vi "bez_daq.vi"() -> ()   [LabVIEW 2019, in "Main.lvlib"]
doc: "Main VI program. \n1. After starting the program, click PowerUP to turn on the calibrator.\n2. The program in Standby can pick the signal values with the use of the keyboard or SetUP mode. \nThe SetUP VI can configure can change the signal type, offset and phase. \n3. Click Operate to go to Operate mode. First 2 Warning message will be shown, then the program will start with Operate mode.\n4. Click Standby to go to standby again, then the program will stop with the DaQ and Operating mode.\n5. Click PowerUP to sotp the program"
uses:
  Main.lvlib
  Tipski Definicii/Kalibrator_Sostojbi.ctl
  Signal/Signal.lvlib
  Tipski Definicii/Keyboard_Sostojbi.ctl
  subVIS/Main_Programs_SubVIs.lvlib
  Tipski Definicii/QMH_Daq_States.ctl
  Polymorphic/Queues.lvlib
  Polymorphic/Enq_DaQ_QMH.vi
  Polymorphic/Enq_Calibrator_QMH.vi
  Polymorphic/Prev_Calibrator_QMH.vi
  Tipski Definicii/check.ctl
  Tipski Definicii/error_handl.ctl
  Tipski Definicii/Signal Values.ctl
  Tipski Definicii/rel_error.ctl
  Tipski Definicii/danger.ctl
  Tipski Definicii/Unit.ctl
  Polymorphic/DeQ_Calibrator_QMH.vi
  Polymorphic/Init_Main.vi
  Polymorphic/Release_Main.vi
  Polymorphic/DaQ_Signal.vi
panel:
  out "AuxA":bool
  out "NormalV":bool
  in  "Knob":dbl(knob) scale=-3.0..3.0 scale format="%#.3g"
  out "Lev_Indikator":string
  out "Desen_Indikator":string
  out "Scope Out":bool
  out "Scope In":bool
  out "AuxAOut":bool
  out "NormalVOut":bool
  in  "V":bool
  in  "Trig":bool
  in  "Tocka":bool
  in  "0":bool
  in  "STBY":bool
  in  "Shift":bool
  in  "SetUP":bool
  in  "Scope":bool
  in  "Save":bool
  in  "Reset":bool
  in  "Power Up":bool
  in  "Plus":bool
  in  "Opr":bool
  in  "Ohm":bool
  in  "NewRef":bool
  in  "Multi":bool
  in  "Meas":bool
  in  "M":bool
  in  "k":bool
  in  "Hz":bool
  in  "F":bool
  in  "Enter":bool
  in  "Earth":bool
  in  "Div":bool
  in  "Conn?":bool
  in  "CE":bool
  in  "C":bool
  in  "Boost":bool
  in  "A":bool
  in  "9":bool
  in  "m":bool
  in  "8":bool
  in  "7":bool
  in  "6":bool
  in  "5":bool
  in  "4":bool
  in  "3":bool
  in  "2":bool
  in  "1":bool
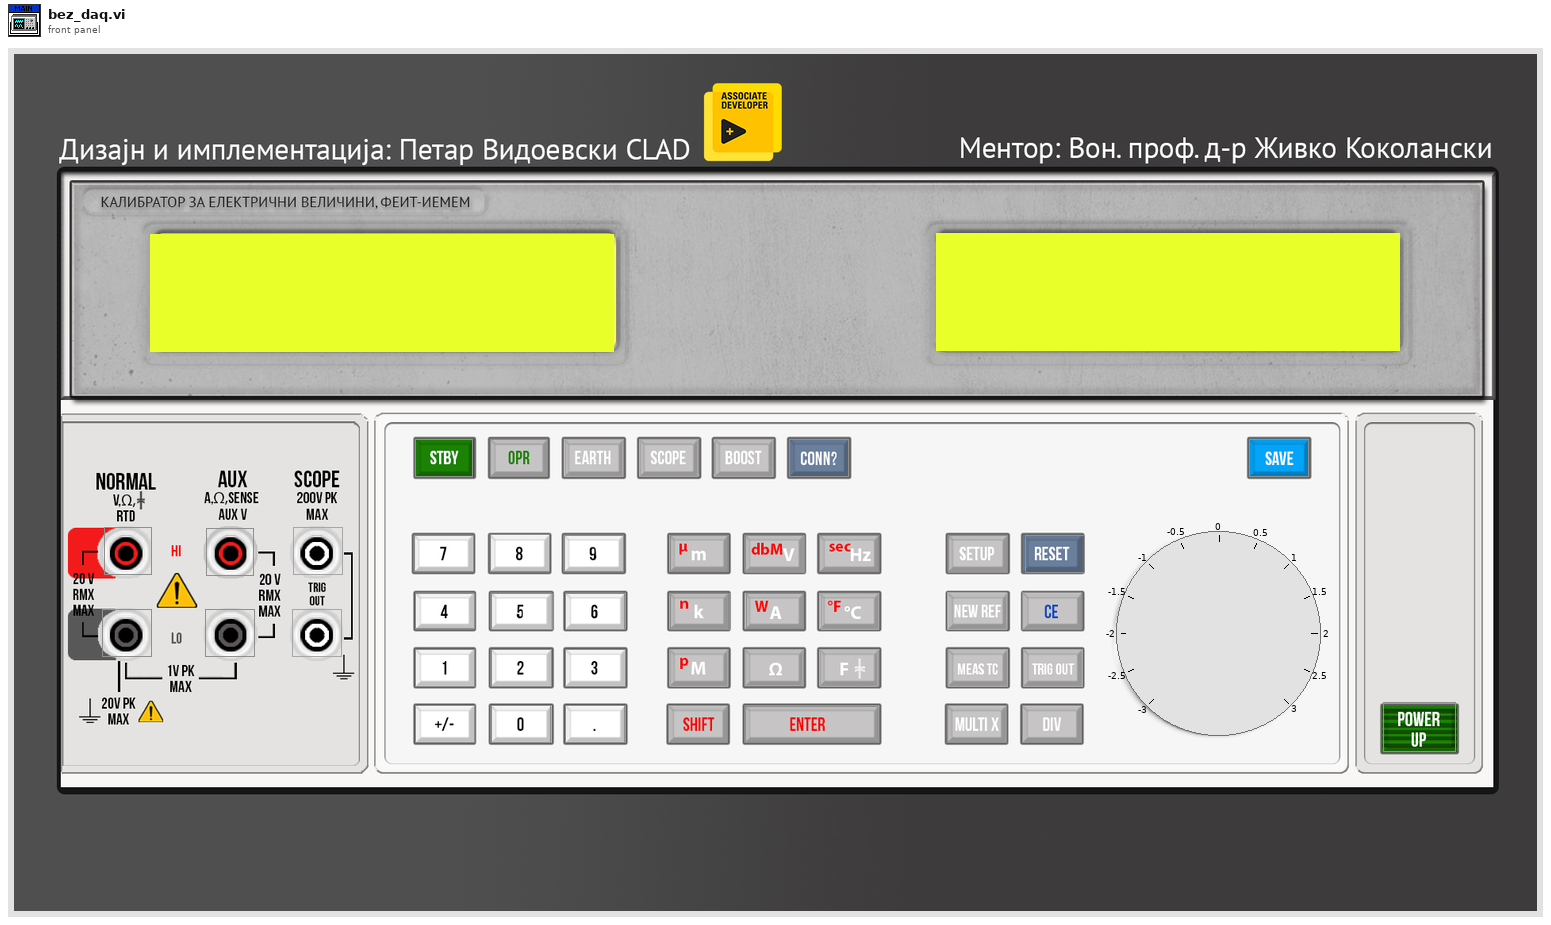
[diagram p1: front panel]
types:
  T1 = cluster{"Calibrator Queue ":refnum<queue>, "ER Refnum":refnum<event-registration>, "User Event in":refnum<user-event>, "QMH Queue ":refnum<queue>, "DaQ Notifier":refnum<notifier>}
  T2 = typedef "Main_program_queues.ctl" = cluster{"Calibrator QMH":refnum<queue>, "DaQ QMH":refnum<queue>, "DaQ":refnum<queue>, "ER":refnum<event-registration>, "User Event":refnum<user-event>}
  T3 = typedef "error_handl.ctl" = enum16{"Init", "Insert Error 1", "Insert Error 2", "Insert Error 3", "Insert Error 4", "Handle Erros"}
  T4 = enum16{"Init", "Init DaQ", "Start", "Output", "Stop", "Delete", "V/A ?"}
  T5 = typedef "Unit.ctl" = enum16{"Init", "Add", "Read"}
  T6 = typedef "rel_error.ctl" = enum16{"Init", "Add String", "Error", "Get Error and Strings", "Reset"}
  T7 = typedef "danger.ctl" = enum16{"Init", "Check"}
  T8 = typedef "check.ctl" = enum16{"Init", "Add dot", "Add +", "Add Shift", "Check", "Reset", "Reset Shift"}
  T9 = typedef "Signal Values.ctl" = enum16{"Init", "Add V/A string", "Add Hz string", "Get Strings and Values", "Reset", "Add Offset", "Add Waveform", "Add Phase"}
  T10 = typedef "Kalibrator_Sostojbi.ctl" = enum16{"Init", "Idle", "Standby", "Operate ", "End"}
  T11 = typedef "Keyboard_Sostojbi.ctl" = enum16{"Init", "Add Number", "Add Decimal", "Add Unit ", "Clear", "Read", "Enter", "CE", "Add Unit Scale", "Check Unit", "Mul", "Div"}
  T12 = cluster{"Amp String":string, "Amp Value":dbl, "Hz Value Out":dbl, "Waveform Out":enum16{"Sine Wave", "Triangle Wave", "Square Wave", "Sawtooth Wave"}, "Offset Out":dbl, "Phase Out":dbl, "Signal String":string, "Signal":waveform(dbl)}
  T13 = cluster{"Voltage":bool, "Current":bool, "Scope":bool}
  T14 = typedef "QMH_Daq_States.ctl" = enum16{"Idle", "Start DaQ", "DaQ", "Generate Message", "Stop DaQ", "End"}
  T15 = enum32{"Invalid", "Standard", "Closed", "Hidden", "Minimized", "Maximized"}
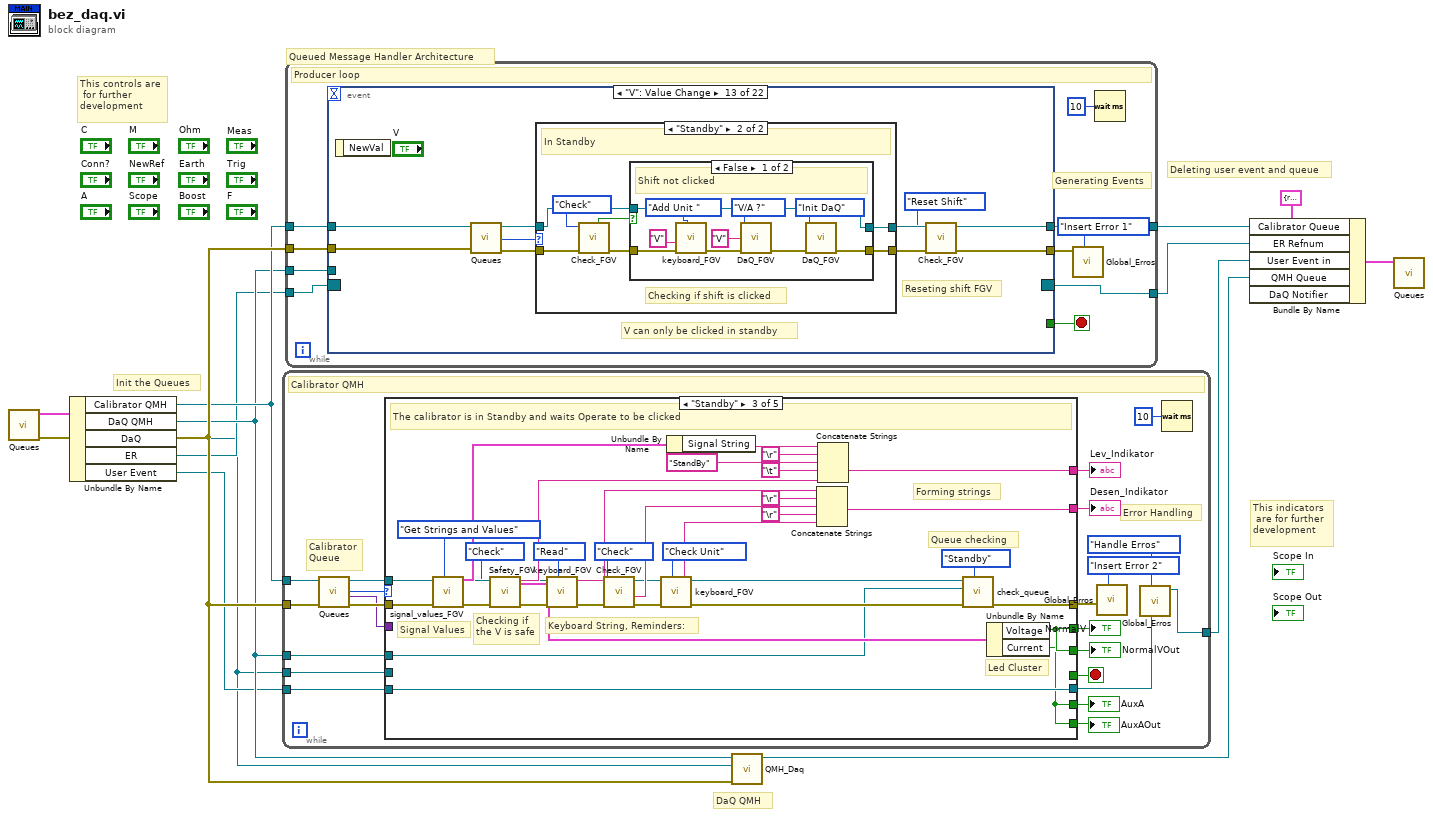
[diagram p0: block diagram]
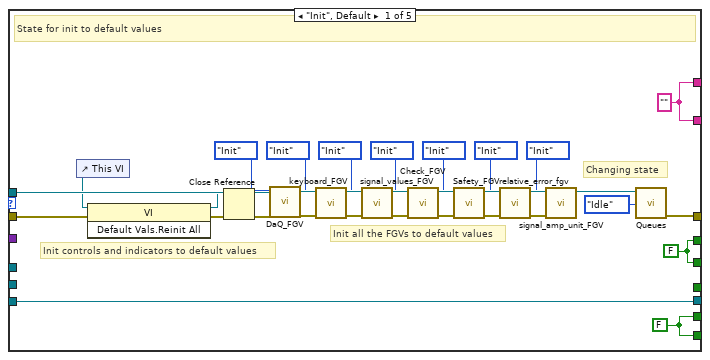
[diagram p2: hidden frame]
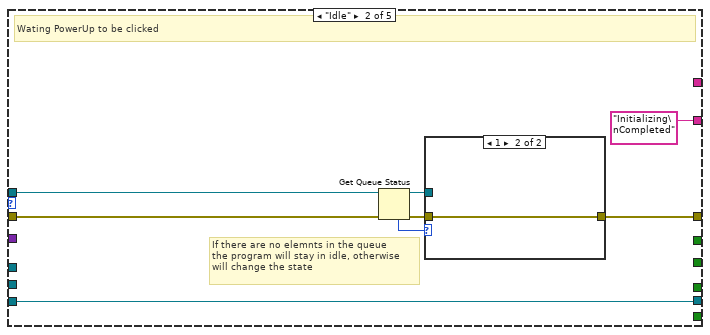
[diagram p3: hidden frame]
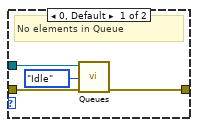
[diagram p4: hidden frame]
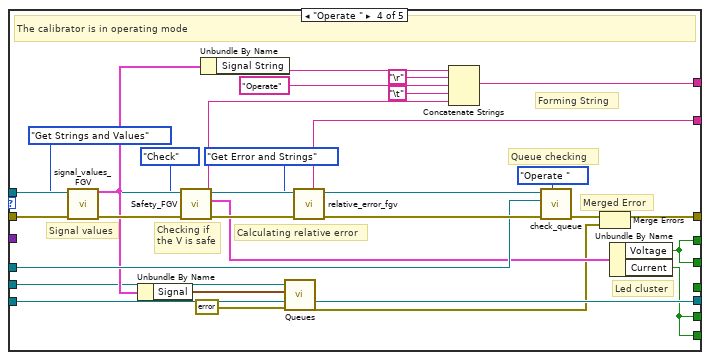
[diagram p5: hidden frame]
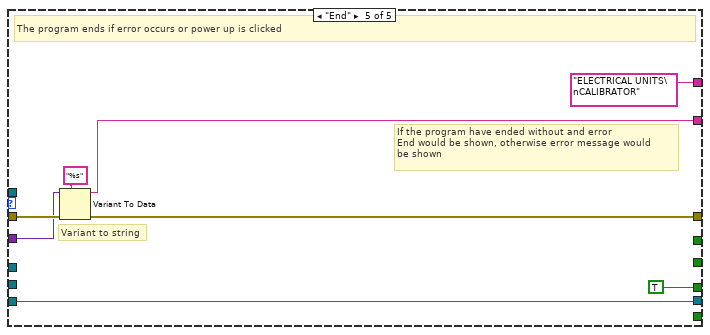
[diagram p6: hidden frame]
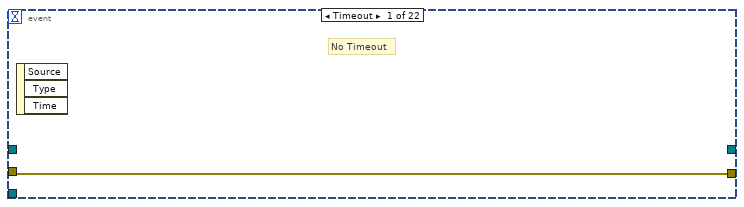
[diagram p7: hidden frame]
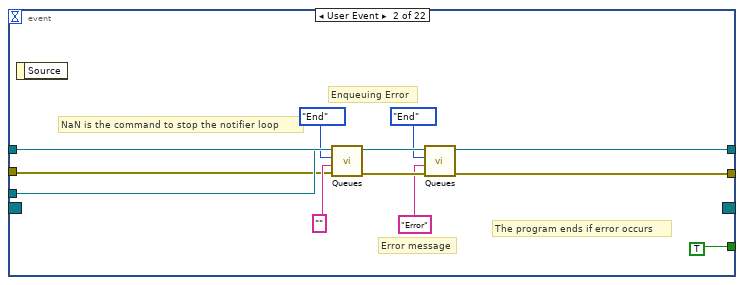
[diagram p8: hidden frame]
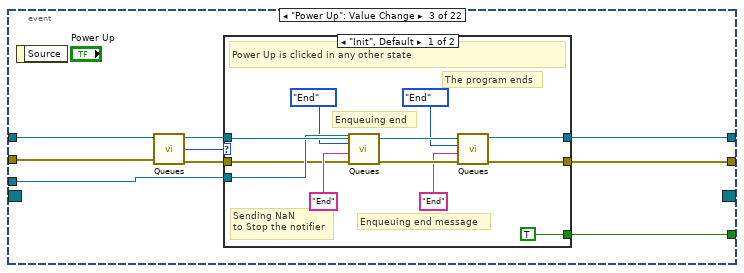
[diagram p9: hidden frame]
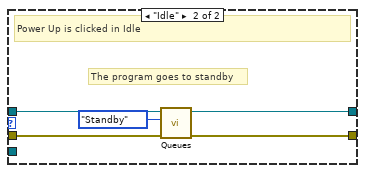
[diagram p10: hidden frame]
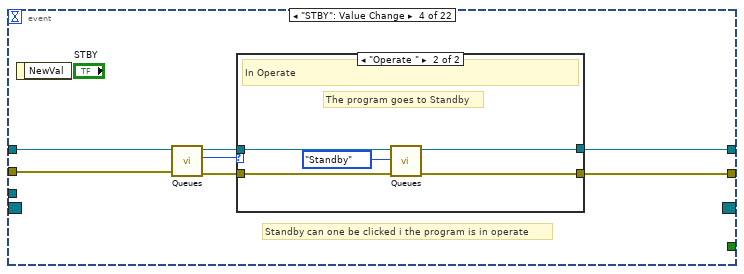
[diagram p11: hidden frame]
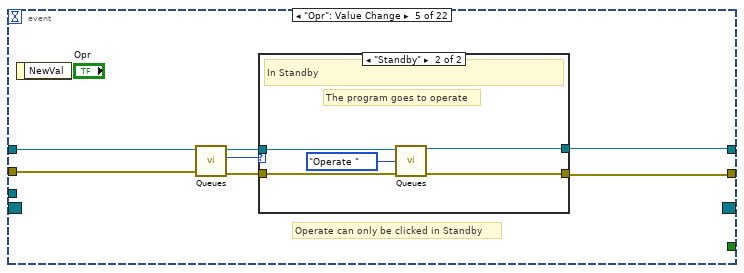
[diagram p13: hidden frame]
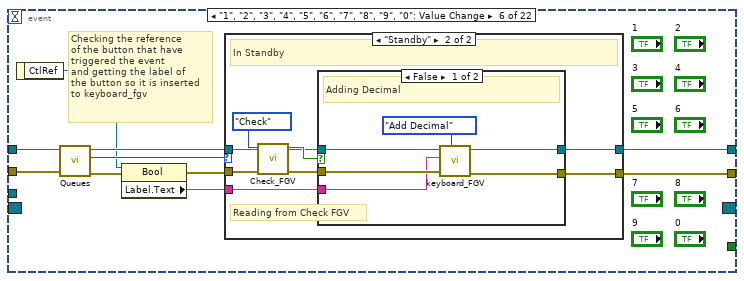
[diagram p15: hidden frame]
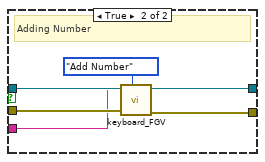
[diagram p17: hidden frame]
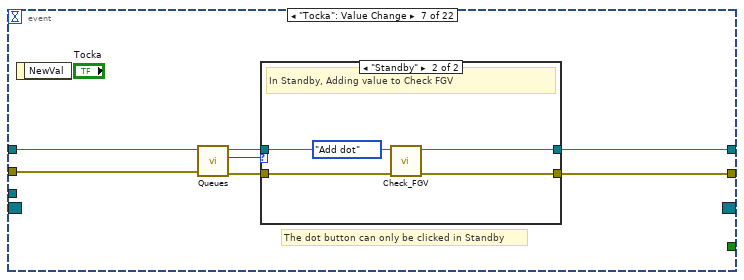
[diagram p18: hidden frame]
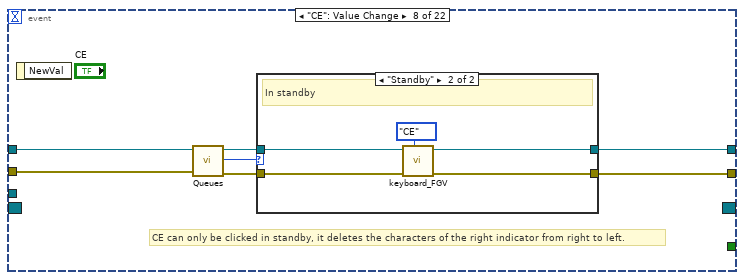
[diagram p20: hidden frame]
diagram:
  # "Init the Queues"
  # "DaQ QMH"
  # "This indicators\n are for further \ndevelopment"
  # "This controls are\n for further \ndevelopment"
  # "Deleting user event and queue"
  # "Queued Message Handler Architecture"
  n1 = call-poly "Queues.vi"() -> ("Error Out"=w13:errorcluster, "Queue Cluster"=w6:T2)  [unwired: 10 in]
  n2 = Unbundle By Name(w6) -> ("Calibrator QMH"=w5:refnum<queue>, "DaQ QMH"=w4:refnum<queue>, "DaQ"=w1:refnum<queue>, "ER"=w3:refnum<event-registration>, "User Event"=w2:refnum<user-event>)
  n3 = while {
    tunnel: w2 -> [w32]
    tunnel: [w28] -> w9
    tunnel: w5 -> [w24]
    tunnel: w4 -> [w30]
    tunnel: w1 -> [w31]
    tunnel: w13 -> [w25]
    stop <- w33 stop-if-true
    # "Calibrator\nQueue"
    # "Error Handling"
    # "Calibrator QMH"
    n4 = call-poly "Queues.vi"("Error In"=w25, "Queue In"=w24) -> ("Error Out"=w23:errorcluster, "Message"=w21:variant, "Instruction"=w22:T10, "Queue Out"=w26:refnum<queue>)  [unwired: 6 in]
    n5 = case shown="\"Standby\"" w22 {
      tunnel: w26 -> [w60 w66 w82 w117 _]
      tunnel: w23 -> [w59 w65 w104 w130 w138]
      tunnel: [w57 "Initializing\nCompleted" ("Desen_Indikator") w98 w125 w135] -> w35
      tunnel: [w57 _ w103 w127 "ELECTRICAL UNITS\nCALIBRATOR" ("Desen_Indikator")] -> w34
      tunnel: [w48 w61 w76 w118 w134] -> w27
      tunnel: [_ _ _ _ TRUE] -> w33
      tunnel: w32 -> [w49 w67 w85 w113 w139]
      tunnel: [w49 w67 w85 w113 w139] -> w29
      tunnel: w30 -> [_ _ w84 w121 _]
      tunnel: w31 -> [_ _ _ w108 _]
      tunnel: w21 -> [_ _ _ _ w136]
      tunnel: [w40 _ w75 w112 _] -> w18
      tunnel: [w40 _ w75 w112 _] -> w17
      tunnel: [w39 _ w74 w110 _] -> w15
      tunnel: [w39 _ w74 w110 _] -> w14
      frame "Init", Default {
        w39 = FALSE ("Current")
        w40 = FALSE ("NormalV")
        w57 = "" ("Desen_Indikator")
        # "Changing state"
        # "Init all the FGVs to default values"
        # "Init controls and indicators to default values"
        # "State for init to default values"
        n6 = control-ref of="This VI"() -> (w58:refnum<vi>)
        n7 = invoke class="VI" method="Default Vals.Reinit All"(reference=w58, error in=w59) -> (reference out=w55:refnum<vi>, error out=w56:errorcluster)  [unwired: 1 in, 1 out]
        n8 = Close Reference(reference=w55, error in (no error)=w56) -> (error out=w38:errorcluster)
        n9 = call "DaQ_FGV.vi"("Error In"=w38, "Action"=T4."Init") -> ("Error Out"=w37:errorcluster)  [unwired: 9 in]
        n10 = call "keyboard_FGV.vi"("Action"=Keyboard_Sostojbi."Init", "Error In"=w37) -> ("Error Out"=w54:errorcluster)  [unwired: 6 in, 3 out]
        n11 = call "signal_values_FGV.vi"("Action"=Signal_Values."Init", "Error In"=w54) -> ("Error Out"=w53:errorcluster)  [unwired: 12 in, 1 out]
        n12 = call "Check_FGV.vi"("Error In"=w53, "Action"=check."Init") -> ("Error Out"=w52:errorcluster)  [unwired: 5 in, 4 out]
        n13 = call "Safety_FGV.vi"("Error In"=w52, "Action"=danger."Init") -> ("Error Out"=w51:errorcluster)  [unwired: 7 in, 2 out]
        n14 = call "relative_error_fgv.vi"("Error In"=w51, "Action"=rel_error."Init") -> ("Error Out"=w42:errorcluster)  [unwired: 5 in, 4 out]
        n15 = call "signal_amp_unit_FGV.vi"("Error In"=w42, "Action"=Unit."Init") -> ()  [unwired: 8 in, 2 out]
        n16 = call-poly "Queues.vi"("Instruction"=Kalibrator_Sostojbi."Idle", "Queue In"=w60) -> ("Error Out"=w48:errorcluster)  [unwired: 8 in, 1 out]
      }
      frame "Idle" {
        # "If there are no elemnts in the queue \nthe program will stay in idle, otherwise \nwill change the state"
        # "Wating PowerUp to be clicked"
        n17 = Get Queue Status(queue=w66, error in (no error)=w65) -> (queue out=w62:refnum<queue>, error out=w63:errorcluster, # elements in queue=w64:i32)  [unwired: 1 in, 5 out]
        n18 = case shown="1" w64 {
          tunnel: w63 -> [w72 w73]
          tunnel: w62 -> [w71 _]
          tunnel: [w69 w73] -> w61
          frame 0, Default {
            # "No elements in Queue"
            n19 = call-poly "Queues.vi"("Error In"=w72, "Instruction"=Kalibrator_Sostojbi."Idle", "Queue In"=w71) -> ("Error Out"=w69:errorcluster)  [unwired: 7 in, 1 out]
          }
          frame 1 {
          }
        }
      }
      frame "Standby" {
        # "Led Cluster"
        # "Queue checking"
        # "Forming strings"
        # "Keyboard String, Reminders:"
        # "Checking if\nthe V is safe"
        # "Signal Values"
        # "The calibrator is in Standby and waits Operate to be clicked"
        n20 = call "signal_values_FGV.vi"("Action"=Signal_Values."Get Strings and Values", "Error In"=w104) -> ("Signal"=w87:T12, "Error Out"=w90:errorcluster)  [unwired: 12 in]
        n21 = call "Safety_FGV.vi"("Error In"=w90, "Action"=danger."Check") -> ("Error Out"=w89:errorcluster, "LED"=w105:T13, "Safetymsg"=w88:string)  [unwired: 7 in]
        n22 = call "keyboard_FGV.vi"("Action"=Keyboard_Sostojbi."Read", "Error In"=w89) -> ("Error Out"=w100:errorcluster, "Indicator Text"=w99:string)  [unwired: 6 in, 2 out]
        n23 = call "Check_FGV.vi"("Error In"=w100, "Action"=check."Check") -> ("Error Out"=w95:errorcluster, "Dot String"=w97:string)  [unwired: 5 in, 3 out]
        n24 = call "keyboard_FGV.vi"("Action"=Keyboard_Sostojbi."Check Unit", "Error In"=w95) -> ("Error Out"=w92:errorcluster, "Unit msg"=w94:string)  [unwired: 6 in, 2 out]
        n25 = Unbundle By Name(w87) -> ("Signal String"=w86:string)
        n26 = Concatenate Strings(w99, "\r", w97, "\r", w94) -> (w98:string)
        n27 = Concatenate Strings(w86, "\r", "StandBy" ("Desen_Indikator"), "\t", w88) -> (w103:string)
        n28 = call "check_queue.vi"("State"=Kalibrator_Sostojbi."Standby", "Error In"=w92, "DaQ QMH"=w84, "Calibrator Queue"=w82) -> ("Error Out"=w76:errorcluster)  [unwired: 7 in]
        n29 = Unbundle By Name(w105) -> ("Voltage"=w75:bool, "Current"=w74:bool)
      }
      frame "Operate " {
        # "Merged Error"
        # "Led cluster"
        # "Forming String"
        # "Queue checking"
        # "Calculating relative error"
        # "Checking if\nthe V is safe"
        # "Signal values"
        # "The calibrator is in operating mode"
        n30 = call "signal_values_FGV.vi"("Action"=Signal_Values."Get Strings and Values", "Error In"=w130) -> ("Signal"=w120:T12, "Error Out"=w128:errorcluster)  [unwired: 12 in]
        n31 = Unbundle By Name(w120) -> ("Signal"=w107:waveform(dbl))
        n32 = call "Safety_FGV.vi"("Error In"=w128, "Action"=danger."Check") -> ("Error Out"=w126:errorcluster, "LED"=w111:T13, "Safetymsg"=w129:string)  [unwired: 7 in]
        n33 = Unbundle By Name(w120) -> ("Signal String"=w124:string)
        n34 = call-poly "Queues.vi"("Error In"=errorcluster {"status"=FALSE, "code"=0, "source"=""} ("error in (no error)"), "Signal"=w107, "Queue In"=w108) -> ("Error Out"=w106:errorcluster)  [unwired: 7 in, 1 out]
        n35 = call "relative_error_fgv.vi"("Error In"=w126, "Action"=rel_error."Get Error and Strings") -> ("Error Out"=w123:errorcluster, "Indicator String"=w125:string)  [unwired: 5 in, 3 out]
        n36 = Concatenate Strings(w124, "\r", "Operate" ("Desen_Indikator"), "\t", w129) -> (w127:string)
        n37 = call "check_queue.vi"("State"=Kalibrator_Sostojbi."Operate ", "Error In"=w123, "DaQ QMH"=w121, "Calibrator Queue"=w117) -> ("Error Out"=w119:errorcluster)  [unwired: 7 in]
        n38 = Merge Errors(w119, w106) -> (w118:errorcluster)
        n39 = Unbundle By Name(w111) -> ("Voltage"=w112:bool, "Current"=w110:bool)
      }
      frame "End" {
        # "If the program have ended without and error\nEnd would be shown, otherwise error message would\nbe shown"
        # "Variant to string"
        # "The program ends if error occurs or power up is clicked"
        n40 = Variant To Data(error in=w138, type="%s", Variant=w136) -> (data=w135:string, error out=w134:errorcluster)
      }
    }
    "Lev_Indikator" <- w34
    "Desen_Indikator" <- w35
    "NormalVOut" <- w17
    "NormalV" <- w18
    "AuxA" <- w15
    "AuxAOut" <- w14
    n41 = call "Global_Erros.vi"("Action"=error_handl."Insert Error 2", "Error Loop2"=w27) -> ()  [unwired: 9 in, 1 out]
    n42 = call "Global_Erros.vi"("User Event In"=w29, "Action"=error_handl."Handle Erros") -> ("User Event Out"=w28:refnum<user-event>)  [unwired: 9 in]
    n43 = Wait (ms)(milliseconds to wait=u32 10) -> ()  [unwired: 1 out]
  }
  n44 = while {
    tunnel: w5 -> [w151]
    tunnel: w13 -> [w146]
    tunnel: [w150] -> w10
    tunnel: w3 -> [w149]
    tunnel: [w147] -> w11
    tunnel: w4 -> [w145]
    stop <- w148 stop-if-true
    # "Generating Events"
    # "Producer loop"
    n45 = event shown="[12] \"V\": Value Change" {
      selector: w149 -> [_ _ _ _ _ _ _ _ _ _ _ _ _ _ _ _ _ _ _ _ _ _]
      dyn-events: [_ _ _ _ _ _ _ _ _ _ _ _ _ _ _ _ _ _ _ _ _ _] -> w150
      timeout: _ -> [_ _ _ _ _ _ _ _ _ _ _ _ _ _ _ _ _ _ _ _ _ _]
      tunnel: w151 -> [_ w163 w167 w191 w205 w224 w250 w263 w276 w299 w313 w328 w355 w383 w414 w440 w465 w493 w503 w521 w544 w560]
      tunnel: w146 -> [w152 w153 w168 w193 w207 w225 w251 w264 w277 w301 w314 w327 w356 w384 w416 w441 w467 w494 w507 w522 w545 w561]
      tunnel: [_ w155 w172 w195 w209 w226 w253 w266 w278 w303 w316 w331 w358 w382 w419 w444 w469 w495 w509 w523 w546 w562] -> w147
      tunnel: [w152 w154 w171 w194 w208 w217 w252 w265 w279 w302 w315 w330 w359 w381 w418 w443 w468 w496 w508 w524 w547 w563] -> w142
      tunnel: [_ TRUE w170 _ _ _ _ _ _ _ _ _ _ _ _ _ _ _ _ _ _ _] -> w148
      tunnel: w145 -> [_ w161 w169 _ _ _ _ _ _ _ _ _ _ _ _ _ _ _ _ _ _ _]
      event Timeout {
        # "No Timeout"
        n46 = event-data() -> ()  [unwired: 1 in, 3 out]
      }
      event User Event {
        # "Enqueuing Error"
        # "Error message"
        # "NaN is the command to stop the notifier loop"
        # "The program ends if error occurs"
        n47 = event-data() -> ()  [unwired: 1 in, 1 out]
        n48 = call-poly "Queues.vi"("Error In"=w153, "Message"="", "Instruction"=QMH_Daq_States."End", "Queue In"=w161) -> ("Error Out"=w158:errorcluster)  [unwired: 6 in, 1 out]
        n49 = call-poly "Queues.vi"("Error In"=w158, "Message"="Error", "Instruction"=Kalibrator_Sostojbi."End", "Queue In"=w163) -> ("Error Out"=w154:errorcluster, "Queue Out"=w155:refnum<queue>)  [unwired: 6 in]
      }
      event "Power Up": Value Change {
        n50 = event-data() -> ()  [unwired: 1 in, 1 out]
        n51 = call-poly "Queues.vi"("Error In"=w168, "Queue In"=w167) -> ("Error Out"=w164:errorcluster, "Instruction"=w165:T10, "Queue Out"=w166:refnum<queue>)  [unwired: 6 in, 1 out]
        n52 = case shown="\"Init\", Default" w165 {
          tunnel: w166 -> [w183 w186]
          tunnel: w164 -> [w173 w188]
          tunnel: [w177 w185] -> w172
          tunnel: [w176 w187] -> w171
          tunnel: [TRUE _] -> w170
          tunnel: w169 -> [w181 _]
          frame "Init", Default {
            # "Enqueuing end"
            # "Enqueuing end message"
            # "Sending NaN\nto Stop the notifier"
            # "The program ends"
            # "Power Up is clicked in any other state"
            n53 = call-poly "Queues.vi"("Error In"=w173, "Message"="End", "Instruction"=QMH_Daq_States."End", "Queue In"=w181) -> ("Error Out"=w178:errorcluster)  [unwired: 6 in, 1 out]
            n54 = call-poly "Queues.vi"("Error In"=w178, "Message"="End", "Instruction"=Kalibrator_Sostojbi."End", "Queue In"=w183) -> ("Error Out"=w176:errorcluster, "Queue Out"=w177:refnum<queue>)  [unwired: 6 in]
          }
          frame "Idle" {
            # "The program goes to standby"
            # "Power Up is clicked in Idle"
            n55 = call-poly "Queues.vi"("Error In"=w188, "Instruction"=Kalibrator_Sostojbi."Standby", "Queue In"=w186) -> ("Error Out"=w187:errorcluster, "Queue Out"=w185:refnum<queue>)  [unwired: 7 in]
          }
        }
      }
      event "STBY": Value Change {
        # "Standby can one be clicked i the program is in operate"
        n56 = event-data() -> ()  [unwired: 1 in, 1 out]
        n57 = call-poly "Queues.vi"("Error In"=w193, "Queue In"=w191) -> ("Error Out"=w192:errorcluster, "Instruction"=w189:T10, "Queue Out"=w190:refnum<queue>)  [unwired: 6 in, 1 out]
        n58 = case shown="\"Operate \"" w189 {
          tunnel: w192 -> [w196 w202]
          tunnel: w190 -> [w197 w200]
          tunnel: [w196 w201] -> w194
          tunnel: [w197 w199] -> w195
          frame "Init", Default {
            # "Not in operate"
          }
          frame "Operate " {
            # "The program goes to Standby"
            # "In Operate"
            n59 = call-poly "Queues.vi"("Error In"=w202, "Instruction"=Kalibrator_Sostojbi."Standby", "Queue In"=w200) -> ("Error Out"=w201:errorcluster, "Queue Out"=w199:refnum<queue>)  [unwired: 7 in]
          }
        }
      }
      event "Opr": Value Change {
        # "Operate can only be clicked in Standby"
        n60 = event-data() -> ()  [unwired: 1 in, 1 out]
        n61 = call-poly "Queues.vi"("Error In"=w207, "Queue In"=w205) -> ("Error Out"=w206:errorcluster, "Instruction"=w203:T10, "Queue Out"=w204:refnum<queue>)  [unwired: 6 in, 1 out]
        n62 = case shown="\"Standby\"" w203 {
          tunnel: w206 -> [w210 w216]
          tunnel: w204 -> [w211 w214]
          tunnel: [w210 w215] -> w208
          tunnel: [w211 w213] -> w209
          frame "Init", Default {
            # "Not in Standby"
          }
          frame "Standby" {
            # "The program goes to operate"
            # "In Standby"
            n63 = call-poly "Queues.vi"("Error In"=w216, "Instruction"=Kalibrator_Sostojbi."Operate ", "Queue In"=w214) -> ("Error Out"=w215:errorcluster, "Queue Out"=w213:refnum<queue>)  [unwired: 7 in]
          }
        }
      }
      event "1", "2", "3", "4", "5", "6", "7", "8", "9", "0": Value Change {
        # "Checking the reference\nof the button that have \ntriggered the event \nand getting the label of \nthe button so it is inserted \nto keyboard_fgv"
        n64 = event-data() -> ("CtlRef"=w219:refnum<vi>)  [unwired: 1 in]
        n65 = call-poly "Queues.vi"("Error In"=w225, "Queue In"=w224) -> ("Error Out"=w221:errorcluster, "Instruction"=w222:T10, "Queue Out"=w223:refnum<queue>)  [unwired: 6 in, 1 out]
        n66 = property class="Bool"(reference=w219, error in=w221) -> (error out=w220:errorcluster, "Label.Text"=w218:string)  [unwired: 1 out]
        n67 = case shown="\"Standby\"" w222 {
          tunnel: w220 -> [w227 w236]
          tunnel: [w227 w233] -> w217
          tunnel: w223 -> [w228 w232]
          tunnel: [w228 w231] -> w226
          tunnel: w218 -> [_ w230]
          frame "Init", Default {
            # "Not in Standby"
          }
          frame "Standby" {
            # "Reading from Check FGV"
            # "In Standby"
            n68 = call "Check_FGV.vi"("Error In"=w236, "Action"=check."Check") -> ("Error Out"=w234:errorcluster, "Number ?"=w235:bool)  [unwired: 5 in, 3 out]
            n69 = case shown="False" w235 {
              tunnel: w234 -> [w241 w246]
              tunnel: [w240 w244] -> w233
              tunnel: w232 -> [w239 w245]
              tunnel: [w239 w245] -> w231
              tunnel: w230 -> [w237 w242]
              frame False {
                # "Adding Decimal"
                n70 = call "keyboard_FGV.vi"("Action"=Keyboard_Sostojbi."Add Decimal", "Error In"=w241, "Decimal"=w237) -> ("Error Out"=w240:errorcluster)  [unwired: 5 in, 3 out]
              }
              frame True {
                # "Adding Number"
                n71 = call "keyboard_FGV.vi"("Action"=Keyboard_Sostojbi."Add Number", "Error In"=w246, "Number"=w242) -> ("Error Out"=w244:errorcluster)  [unwired: 5 in, 3 out]
              }
            }
          }
        }
      }
      event "Tocka": Value Change {
        # "The dot button can only be clicked in Standby"
        n72 = event-data() -> ()  [unwired: 1 in, 1 out]
        n73 = call-poly "Queues.vi"("Error In"=w251, "Queue In"=w250) -> ("Error Out"=w247:errorcluster, "Instruction"=w248:T10, "Queue Out"=w249:refnum<queue>)  [unwired: 6 in, 1 out]
        n74 = case shown="\"Standby\"" w248 {
          tunnel: w247 -> [w254 w257]
          tunnel: [w255 w259] -> w253
          tunnel: w249 -> [w255 w259]
          tunnel: [w254 w258] -> w252
          frame "Init", Default {
            # "Not in Standby"
          }
          frame "Standby" {
            # "In Standby, Adding value to Check FGV"
            n75 = call "Check_FGV.vi"("Error In"=w257, "Action"=check."Add dot") -> ("Error Out"=w258:errorcluster)  [unwired: 5 in, 4 out]
          }
        }
      }
      event "CE": Value Change {
        # "CE can only be clicked in standby, it deletes the characters of the right indicator from right to left."
        n76 = event-data() -> ()  [unwired: 1 in, 1 out]
        n77 = call-poly "Queues.vi"("Error In"=w264, "Queue In"=w263) -> ("Error Out"=w260:errorcluster, "Instruction"=w261:T10, "Queue Out"=w262:refnum<queue>)  [unwired: 6 in, 1 out]
        n78 = case shown="\"Standby\"" w261 {
          tunnel: w260 -> [w267 w272]
          tunnel: w262 -> [w268 w271]
          tunnel: [w268 w271] -> w266
          tunnel: [w267 w270] -> w265
          frame "Init", Default {
            # "Not in standby"
          }
          frame "Standby" {
            # "In standby"
            n79 = call "keyboard_FGV.vi"("Action"=Keyboard_Sostojbi."CE", "Error In"=w272) -> ("Error Out"=w270:errorcluster)  [unwired: 6 in, 3 out]
          }
        }
      }
      event "Enter": Value Change {
        # "Enter can only be clicked if the program is in Standby and value electrical unit is picked"
        n80 = event-data() -> ()  [unwired: 1 in, 1 out]
        n81 = call-poly "Queues.vi"("Error In"=w277, "Queue In"=w276) -> ("Error Out"=w274:errorcluster, "Instruction"=w273:T10, "Queue Out"=w275:refnum<queue>)  [unwired: 6 in, 1 out]
        n82 = case shown="\"Standby\"" w273 {
          tunnel: w274 -> [w280 w287]
          tunnel: w275 -> [w281 w284]
          tunnel: [w280 w288] -> w279
          tunnel: [w281 w282] -> w278
          frame "Init", Default {
            # "Not in Standby"
          }
          frame "Standby" {
            # "Checking if unit is enterd"
            # "In Standby"
            n83 = call "keyboard_FGV.vi"("Action"=Keyboard_Sostojbi."Check Unit", "Error In"=w287) -> ("Error Out"=w283:errorcluster, "Unit"=w285:bool)  [unwired: 6 in, 2 out]
            n84 = case shown="True" w285 {
              tunnel: [w293 w295] -> w288
              tunnel: [w289 w296] -> w282
              tunnel: w284 -> [w289 w296]
              tunnel: w283 -> [w290 w295]
              frame False {
                # "Unit is entered"
                n85 = call "keyboard_FGV.vi"("Action"=Keyboard_Sostojbi."Enter", "Error In"=w290) -> ("Error Out"=w294:errorcluster)  [unwired: 6 in, 3 out]
                n86 = call "keyboard_FGV.vi"("Action"=Keyboard_Sostojbi."Clear", "Error In"=w294) -> ("Error Out"=w293:errorcluster)  [unwired: 6 in, 3 out]
              }
              frame True {
                # "No unit entered"
              }
            }
          }
        }
      }
      event "Plus": Value Change {
        # "The plus button can only be clicked in Standby, it is used to change the polarity of the voltage"
        n87 = event-data() -> ()  [unwired: 1 in, 1 out]
        n88 = call-poly "Queues.vi"("Error In"=w301, "Queue In"=w299) -> ("Error Out"=w300:errorcluster, "Instruction"=w297:T10, "Queue Out"=w298:refnum<queue>)  [unwired: 6 in, 1 out]
        n89 = case shown="\"Standby\"" w297 {
          tunnel: [w305 w308] -> w303
          tunnel: w298 -> [w305 w308]
          tunnel: w300 -> [w304 w309]
          tunnel: [w304 w307] -> w302
          frame "Init", Default {
            # "Not in Standby"
          }
          frame "Standby" {
            # "Adding value to Check FGV"
            # "In Standby"
            n90 = call "Check_FGV.vi"("Error In"=w309, "Action"=check."Add +") -> ("Error Out"=w307:errorcluster)  [unwired: 5 in, 4 out]
          }
        }
      }
      event "Shift": Value Change {
        # "Shift can only be clicked in Standby. If shift is clicked the usser can pick the \nsecondary options of the units keyboard"
        n91 = event-data() -> ()  [unwired: 1 in, 1 out]
        n92 = call-poly "Queues.vi"("Error In"=w314, "Queue In"=w313) -> ("Error Out"=w311:errorcluster, "Instruction"=w310:T10, "Queue Out"=w312:refnum<queue>)  [unwired: 6 in, 1 out]
        n93 = case shown="\"Standby\"" w310 {
          tunnel: w311 -> [w317 w322]
          tunnel: w312 -> [w318 w321]
          tunnel: [w318 w321] -> w316
          tunnel: [w317 w320] -> w315
          frame "Init", Default {
            # "Not in Standby"
          }
          frame "Standby" {
            # "Adding value to the Shift FGV"
            # "In Standby"
            n94 = call "Check_FGV.vi"("Error In"=w322, "Action"=check."Add Shift") -> ("Error Out"=w320:errorcluster)  [unwired: 5 in, 4 out]
          }
        }
      }
      event "m": Value Change {
        # "Reset shift FGV"
        # "m can only be clicked in standby"
        n95 = event-data() -> ()  [unwired: 1 in, 1 out]
        n96 = call-poly "Queues.vi"("Error In"=w327, "Queue In"=w328) -> ("Error Out"=w324:errorcluster, "Instruction"=w326:T10, "Queue Out"=w325:refnum<queue>)  [unwired: 6 in, 1 out]
        n97 = case shown="\"Standby\"" w326 {
          tunnel: w325 -> [w333 w337]
          tunnel: w324 -> [w332 w340]
          tunnel: [w333 w336] -> w331
          tunnel: [w332 w335] -> w329
          frame "Init", Default {
            # "Not in Standby"
          }
          frame "Standby" {
            # "Checking if shift is clicked before m"
            # "In Standby"
            n98 = call "Check_FGV.vi"("Error In"=w340, "Action"=check."Check") -> ("Error Out"=w338:errorcluster, "Shift ?"=w339:bool)  [unwired: 5 in, 3 out]
            n99 = case shown="False" w339 {
              tunnel: w338 -> [w345 w348]
              tunnel: w337 -> [w342 w347]
              tunnel: [w342 w347] -> w336
              tunnel: [w341 w346] -> w335
              frame False {
                # "No shift clicked"
                n100 = call "keyboard_FGV.vi"("Unit scale"="m", "Action"=Keyboard_Sostojbi."Add Unit Scale", "Error In"=w345) -> ("Error Out"=w341:errorcluster)  [unwired: 5 in, 3 out]
              }
              frame True {
                # "Shift clicked"
                n101 = call "keyboard_FGV.vi"("Unit scale"="micro", "Action"=Keyboard_Sostojbi."Add Unit Scale", "Error In"=w348) -> ("Error Out"=w346:errorcluster)  [unwired: 5 in, 3 out]
              }
            }
          }
        }
        n102 = call "Check_FGV.vi"("Error In"=w329, "Action"=check."Reset Shift") -> ("Error Out"=w330:errorcluster)  [unwired: 5 in, 4 out]
      }
      event "V": Value Change {
        # "Reseting shift FGV"
        # "V can only be clicked in standby"
        n103 = event-data() -> ()  [unwired: 1 in, 1 out]
        n104 = call-poly "Queues.vi"("Error In"=w356, "Queue In"=w355) -> ("Error Out"=w353:errorcluster, "Instruction"=w352:T10, "Queue Out"=w354:refnum<queue>)  [unwired: 6 in, 1 out]
        n105 = case shown="\"Standby\"" w352 {
          tunnel: w354 -> [w361 w365]
          tunnel: w353 -> [w360 w368]
          tunnel: [w361 w364] -> w358
          tunnel: [w360 w363] -> w357
          frame "Init", Default {
            # "Not in standby"
          }
          frame "Standby" {
            # "Checking if shift is clicked"
            # "In Standby"
            n106 = call "Check_FGV.vi"("Error In"=w368, "Action"=check."Check") -> ("Error Out"=w366:errorcluster, "Shift ?"=w367:bool)  [unwired: 5 in, 3 out]
            n107 = case shown="False" w367 {
              tunnel: w366 -> [w378 w379]
              tunnel: w365 -> [w375 w380]
              tunnel: [w375 w380] -> w364
              tunnel: [w370 w379] -> w363
              frame False {
                # "Shift not clicked"
                n108 = call "keyboard_FGV.vi"("Action"=Keyboard_Sostojbi."Add Unit ", "Error In"=w378, "Unit"="V" ("Unit scale")) -> ("Error Out"=w374:errorcluster)  [unwired: 5 in, 3 out]
                n109 = call "DaQ_FGV.vi"("Error In"=w374, "V/A?"="V", "Action"=T4."V/A ?") -> ("Error Out"=w371:errorcluster)  [unwired: 8 in]
                n110 = call "DaQ_FGV.vi"("Error In"=w371, "Action"=T4."Init DaQ") -> ("Error Out"=w370:errorcluster)  [unwired: 9 in]
              }
              frame True {
                # "Shift clicked"
              }
            }
          }
        }
        n111 = call "Check_FGV.vi"("Error In"=w357, "Action"=check."Reset Shift") -> ("Error Out"=w359:errorcluster)  [unwired: 5 in, 4 out]
      }
      event "A": Value Change {
        # "Reseting shift FGV"
        # "A can only be clicked in standby"
        n112 = event-data() -> ()  [unwired: 1 in, 1 out]
        n113 = call-poly "Queues.vi"("Error In"=w384, "Queue In"=w383) -> ("Error Out"=w387:errorcluster, "Instruction"=w386:T10, "Queue Out"=w388:refnum<queue>)  [unwired: 6 in, 1 out]
        n114 = case shown="\"Standby\"" w386 {
          tunnel: w388 -> [w391 w395]
          tunnel: w387 -> [w390 w398]
          tunnel: [w391 w394] -> w382
          tunnel: [w390 w393] -> w389
          frame "Init", Default {
            # "Not in standby"
          }
          frame "Standby" {
            # "Checking if shift is clicked"
            # "In Standby"
            n115 = call "Check_FGV.vi"("Error In"=w398, "Action"=check."Check") -> ("Error Out"=w396:errorcluster, "Shift ?"=w397:bool)  [unwired: 5 in, 3 out]
            n116 = case shown="False" w397 {
              tunnel: w396 -> [w408 w409]
              tunnel: w395 -> [w405 w410]
              tunnel: [w405 w410] -> w394
              tunnel: [w400 w409] -> w393
              frame False {
                # "Shift not clicked"
                n117 = call "keyboard_FGV.vi"("Action"=Keyboard_Sostojbi."Add Unit ", "Error In"=w408, "Unit"="A" ("Unit scale")) -> ("Error Out"=w404:errorcluster)  [unwired: 5 in, 3 out]
                n118 = call "DaQ_FGV.vi"("Error In"=w404, "V/A?"="A", "Action"=T4."V/A ?") -> ("Error Out"=w401:errorcluster)  [unwired: 8 in]
                n119 = call "DaQ_FGV.vi"("Error In"=w401, "Action"=T4."Init DaQ") -> ("Error Out"=w400:errorcluster)  [unwired: 9 in]
              }
              frame True {
                # "Shift clicked"
              }
            }
          }
        }
        n120 = call "Check_FGV.vi"("Error In"=w389, "Action"=check."Reset Shift") -> ("Error Out"=w381:errorcluster)  [unwired: 5 in, 4 out]
      }
      event "Hz": Value Change {
        # "Reseting shift FGV"
        # "Hz can only be clicked in Standby"
        n121 = event-data() -> ()  [unwired: 1 in, 1 out]
        n122 = call-poly "Queues.vi"("Error In"=w416, "Queue In"=w414) -> ("Error Out"=w415:errorcluster, "Instruction"=w412:T10, "Queue Out"=w413:refnum<queue>)  [unwired: 6 in, 1 out]
        n123 = case shown="\"Standby\"" w412 {
          tunnel: w413 -> [w421 w425]
          tunnel: w415 -> [w420 w428]
          tunnel: [w421 w424] -> w419
          tunnel: [w420 w423] -> w417
          frame "Init", Default {
            # "Not in standby"
          }
          frame "Standby" {
            # "Checking if shift is clicked"
            # "In standby"
            n124 = call "Check_FGV.vi"("Error In"=w428, "Action"=check."Check") -> ("Error Out"=w426:errorcluster, "Shift ?"=w427:bool)  [unwired: 5 in, 3 out]
            n125 = case shown="False" w427 {
              tunnel: w426 -> [w433 w434]
              tunnel: w425 -> [w431 w435]
              tunnel: [w431 w435] -> w424
              tunnel: [w430 w434] -> w423
              frame False {
                # "Shift was not clicked"
                n126 = call "keyboard_FGV.vi"("Action"=Keyboard_Sostojbi."Add Unit ", "Error In"=w433, "Unit"="Hz" ("Unit scale")) -> ("Error Out"=w430:errorcluster)  [unwired: 5 in, 3 out]
              }
              frame True {
                # "Shift clicked"
              }
            }
          }
        }
        n127 = call "Check_FGV.vi"("Error In"=w417, "Action"=check."Reset Shift") -> ("Error Out"=w418:errorcluster)  [unwired: 5 in, 4 out]
      }
      event "k": Value Change {
        # "Reseting shfit FGV"
        # "k can only be clicked in standby"
        n128 = event-data() -> ()  [unwired: 1 in, 1 out]
        n129 = call-poly "Queues.vi"("Error In"=w441, "Queue In"=w440) -> ("Error Out"=w438:errorcluster, "Instruction"=w437:T10, "Queue Out"=w439:refnum<queue>)  [unwired: 6 in, 1 out]
        n130 = case shown="\"Standby\"" w437 {
          tunnel: w439 -> [w446 w450]
          tunnel: w438 -> [w445 w453]
          tunnel: [w446 w449] -> w444
          tunnel: [w445 w448] -> w442
          frame "Init", Default {
            # "Not in standby"
          }
          frame "Standby" {
            # "Checking if shift was clicked"
            # "In standby"
            n131 = call "Check_FGV.vi"("Error In"=w453, "Action"=check."Check") -> ("Error Out"=w451:errorcluster, "Shift ?"=w452:bool)  [unwired: 5 in, 3 out]
            n132 = case shown="False" w452 {
              tunnel: w451 -> [w456 w459]
              tunnel: w450 -> [w455 w460]
              tunnel: [w455 w460] -> w449
              tunnel: [w454 w459] -> w448
              frame False {
                # "Shift Not clicked"
                n133 = call "keyboard_FGV.vi"("Unit scale"="k", "Action"=Keyboard_Sostojbi."Add Unit Scale", "Error In"=w456) -> ("Error Out"=w454:errorcluster)  [unwired: 5 in, 3 out]
              }
              frame True {
                # "Shift clicked"
              }
            }
          }
        }
        n134 = call "Check_FGV.vi"("Error In"=w442, "Action"=check."Reset Shift") -> ("Error Out"=w443:errorcluster)  [unwired: 5 in, 4 out]
      }
      event "Reset": Value Change {
        # "Reset can only be clicked if the program is not in idle"
        n135 = event-data() -> ()  [unwired: 1 in, 1 out]
        n136 = call-poly "Queues.vi"("Error In"=w467, "Queue In"=w465) -> ("Error Out"=w466:errorcluster, "Instruction"=w462:T10, "Queue Out"=w464:refnum<queue>)  [unwired: 6 in, 1 out]
        n137 = Equal?(x=w462, y=Kalibrator_Sostojbi."Idle") -> (x = y?=w463:bool)
        n138 = case shown="False" w463 {
          tunnel: [w477 w489] -> w469
          tunnel: w464 -> [w474 w489]
          tunnel: w466 -> [w480 w488]
          tunnel: [w476 w488] -> w468
          frame False {
            # "Reseting keyboard FGV, and signal values FGV"
            # "Not in Idle"
            n139 = call "keyboard_FGV.vi"("Action"=Keyboard_Sostojbi."Clear", "Error In"=w480) -> ("Error Out"=w479:errorcluster)  [unwired: 6 in, 3 out]
            n140 = call "signal_values_FGV.vi"("Action"=Signal_Values."Reset", "Error In"=w479) -> ("Error Out"=w475:errorcluster)  [unwired: 12 in, 1 out]
            n141 = call-poly "Queues.vi"("Error In"=w475, "Queue In"=w474) -> ("Error Out"=w472:errorcluster, "Instruction"=w471:T10, "Queue Out"=w473:refnum<queue>)  [unwired: 6 in, 1 out]
            n142 = case shown="\"Operate \", Default" w471 {
              tunnel: w472 -> [w485 w487]
              tunnel: w473 -> [w483 w486]
              tunnel: [w482 w486] -> w477
              tunnel: [w484 w487] -> w476
              frame "Operate ", Default {
                # "The program goes\nto Stadnby"
                # "Clicked in Operate"
                n143 = call-poly "Queues.vi"("Error In"=w485, "Instruction"=Kalibrator_Sostojbi."Standby", "Queue In"=w483) -> ("Error Out"=w484:errorcluster, "Queue Out"=w482:refnum<queue>)  [unwired: 7 in]
              }
              frame "Standby" {
                # "The program stays in\nstandby"
                # "Reset clicked in standby"
              }
            }
          }
          frame True {
            # "In idle"
          }
        }
      }
      event "Multi": Value Change {
        # "Multi, can only be clicekd in Standby, and is used to \nmultiply the keyboard value by 10."
        n144 = event-data() -> ()  [unwired: 1 in, 1 out]
        n145 = call-poly "Queues.vi"("Error In"=w494, "Queue In"=w493) -> ("Error Out"=w491:errorcluster, "Instruction"=w490:T10, "Queue Out"=w492:refnum<queue>)  [unwired: 6 in, 1 out]
        n146 = case shown="\"Standby\"" w490 {
          tunnel: [w497 w499] -> w496
          tunnel: w492 -> [w498 w501]
          tunnel: [w498 w501] -> w495
          tunnel: w491 -> [w497 w500]
          frame "Init", Default {
            # "Not in standby"
          }
          frame "Standby" {
            # "In standby"
            n147 = call "keyboard_FGV.vi"("Action"=Keyboard_Sostojbi."Mul", "Error In"=w500) -> ("Error Out"=w499:errorcluster)  [unwired: 6 in, 3 out]
          }
        }
      }
      event "Div": Value Change {
        # "Div, can only be clicekd in Standby, and is used to \ndivide the keyboard value by 10."
        n148 = event-data() -> ()  [unwired: 1 in, 1 out]
        n149 = call-poly "Queues.vi"("Error In"=w507, "Queue In"=w503) -> ("Error Out"=w506:errorcluster, "Instruction"=w505:T10, "Queue Out"=w504:refnum<queue>)  [unwired: 6 in, 1 out]
        n150 = case shown="\"Standby\"" w505 {
          tunnel: [w510 w514] -> w508
          tunnel: w506 -> [w510 w513]
          tunnel: w504 -> [w511 w512]
          tunnel: [w511 w512] -> w509
          frame "Init", Default {
            # "Not in Standby"
          }
          frame "Standby" {
            # "Standby"
            n151 = call "keyboard_FGV.vi"("Action"=Keyboard_Sostojbi."Div", "Error In"=w513) -> ("Error Out"=w514:errorcluster)  [unwired: 6 in, 3 out]
          }
        }
      }
      event "SetUP": Value Change {
        # "Opening  \nMaximized\nFront Panel"
        # "Minimazing the main VI"
        # "SetUp can only be clicked if the program is not in idle\nThen the SetUP VI will be opened"
        n152 = event-data() -> ()  [unwired: 1 in, 1 out]
        n153 = call-poly "Queues.vi"("Error In"=w522, "Queue In"=w521) -> ("Error Out"=w516:errorcluster, "Instruction"=w518:T10, "Queue Out"=w520:refnum<queue>)  [unwired: 6 in, 1 out]
        n154 = Equal?(x=w518, y=Kalibrator_Sostojbi."Idle") -> (x = y?=w519:bool)
        n155 = case shown="False" w519 {
          tunnel: w516 -> [w529 w539]
          tunnel: [w526 w539] -> w524
          tunnel: w520 -> [w534 w540]
          tunnel: [w534 w540] -> w523
          frame False {
            # "Run Vi"
            # "SetUP reference"
            # "Not in Idle"
            n156 = control-ref of="This VI"() -> (w532:refnum<vi>)
            n157 = property class="VI"(reference=w532, error in=w529, "FP.State"=T15."Minimized" ("Front Panel Window:State")) -> (reference out=w533:refnum<vi>, error out=w531:errorcluster)
            n158 = Close Reference(reference=w533, error in (no error)=w531) -> (error out=w528:errorcluster)
            n159 = vi-ref "Setup.vi"() -> (w538:refnum<vi>)
            n160 = invoke class="VI" method="FP.Open"(reference=w538, error in=w528, "Activate"=TRUE ("Activate?"), "State"=T15."Maximized") -> (reference out=w536:refnum<vi>, error out=w535:errorcluster)  [unwired: 1 in, 3 out]
            n161 = invoke class="VI" method="Run VI"(reference=w536, error in=w535, "Auto Dispose Ref"=TRUE ("Auto Dispose Reference")) -> (error out=w526:errorcluster)  [unwired: 2 in, 4 out]
          }
          frame True {
            # "In Idle"
          }
        }
      }
      event "Knob": Value Change {
        n162 = event-data() -> ()  [unwired: 1 in, 1 out]
        n163 = call-poly "Queues.vi"("Error In"=w545, "Queue In"=w544) -> ("Error Out"=w542:errorcluster, "Instruction"=w541:T10, "Queue Out"=w543:refnum<queue>)  [unwired: 6 in, 1 out]
        n164 = case shown="\"Operate \"" w541 {
          tunnel: [w548 w553] -> w547
          tunnel: w543 -> [w549 w552]
          tunnel: [w549 w552] -> w546
          tunnel: w542 -> [w548 w551]
          frame "Init", Default {
            # "Not In operate"
          }
          frame "Operate " {
            # "In Operate"
            n165 = call "relative_error_fgv.vi"("Error In"=w551, "Knob"="Knob", "Action"=rel_error."Error") -> ("Error Out"=w553:errorcluster)  [unwired: 4 in, 4 out]
          }
        }
      }
      event "Save": Value Change {
        # "Save can only be clicked in operate and it will open the Save VI where the user can enter the data for the table"
        n166 = event-data() -> ()  [unwired: 1 in, 1 out]
        n167 = call-poly "Queues.vi"("Error In"=w561, "Queue In"=w560) -> ("Error Out"=w555:errorcluster, "Instruction"=w557:T10, "Queue Out"=w559:refnum<queue>)  [unwired: 6 in, 1 out]
        n168 = Equal?(x=w557, y=Kalibrator_Sostojbi."Operate ") -> (x = y?=w558:bool)
        n169 = case shown="True" w558 {
          tunnel: w555 -> [w564 w571]
          tunnel: [w564 w567] -> w563
          tunnel: w559 -> [w565 w569]
          tunnel: [w565 w569] -> w562
          frame False {
            # "Not in operate"
          }
          frame True {
            # "Opening  \nMaximized\nFront Panel"
            # "Save reference"
            # "In operate"
            n170 = control-ref of="This VI"() -> (w574:refnum<vi>)
            n171 = property class="VI"(reference=w574, error in=w571, "FP.State"=T15."Minimized" ("Front Panel Window:State")) -> (reference out=w575:refnum<vi>, error out=w573:errorcluster)
            n172 = Close Reference(reference=w575, error in (no error)=w573) -> (error out=w570:errorcluster)
            n173 = vi-ref "Save.vi"() -> (w579:refnum<vi>)
            n174 = invoke class="VI" method="FP.Open"(reference=w579, error in=w570, "Activate"=TRUE ("Activate?"), "State"=T15."Maximized") -> (reference out=w577:refnum<vi>, error out=w576:errorcluster)  [unwired: 1 in, 3 out]
            n175 = invoke class="VI" method="Run VI"(reference=w577, error in=w576, "Auto Dispose Ref"=TRUE ("Auto Dispose Reference")) -> (error out=w567:errorcluster)  [unwired: 2 in, 4 out]
          }
        }
      }
    }
    n176 = call "Global_Erros.vi"("Action"=error_handl."Insert Error 1", "Error Loop 1"=w142) -> ()  [unwired: 9 in, 1 out]
    n177 = Wait (ms)(milliseconds to wait=u32 10) -> ()  [unwired: 1 out]
  }
  n178 = call "QMH_Daq.vi"("Error In"=w13, "DaQ Queue In"=w1, "QMH Queue"=w4) -> ("QMH Queue Out"=w8:refnum<queue>)  [unwired: 7 in, 1 out]
  n179 = Bundle By Name(cluster=T1 {"Calibrator Queue "=refnum, "ER Refnum"=refnum, "User Event in"=refnum, "QMH Queue "=refnum, "DaQ Notifier"=refnum} ("Input Cluster"), "Calibrator Queue"=w11, "ER Refnum"=w10, "User Event in"=w9, "QMH Queue"=w8) -> (w7:T1)  [unwired: 1 in]
  n180 = call-poly "Queues.vi"("Queues"=w7) -> ()  [unwired: 11 in]
